vi "Reset Front Panel Origin.vi"(8 "Error In":errorcluster, 11 "VI Reference":refnum<vi>) -> (0 "Error Out":errorcluster)   [LabVIEW 2022 SP3]
doc: "This VI sets the front panel origin"
uses:
  <vilib>/Utility/miscctls.llb/LVPointTypeDef.ctl
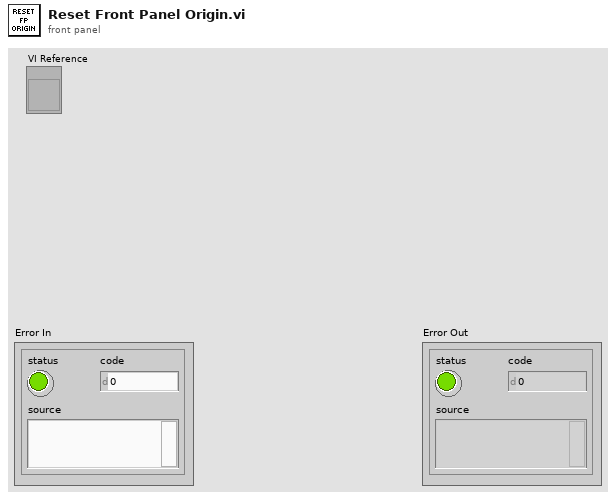
[diagram p1: front panel]
types:
  T1 = typedef "LVPointTypeDef.ctl" = cluster{"Horizontal":i16, "Vertical":i16}
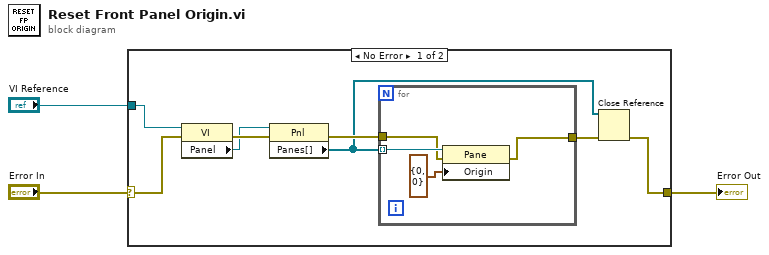
[diagram p0: block diagram]
diagram:
  n1 = case shown="No Error" "Error In" {
    selector: "Error In" -> [w10 w16]
    tunnel: [w4 w16] -> w2
    tunnel: "VI Reference" -> [w11 _]
    frame No Error {
      n2 = property class="VI"(reference=w11, error in=w10) -> (error out=w9:errorcluster, "Panel"=w8:refnum<vi>)  [unwired: 1 out]
      n3 = property class="Pnl"(reference=w8, error in=w9) -> (error out=w7:errorcluster, "Panes[]"=w5:refnum<vi>[])  [unwired: 1 out]
      n4 = for {
        tunnel: w5 -> [w15] mode=indexing
        tunnel: w7 -> [w14]
        tunnel: [w13] -> w6
        n5 = property class="Pane"(reference=w15, error in=w14, "Origin"=T1 {"Horizontal"=0, "Vertical"=0}) -> (error out=w13:errorcluster)  [unwired: 1 out]
      }
      n6 = Close Reference(reference=w5, error in (no error)=w6) -> (error out=w4:errorcluster)
    }
    frame Error {
    }
  }
  "Error Out" <- w2
